vi "write_metadata_attributes.vi"(5 "Group ID":string, 6 "error in (no error)":errorcluster, 8 "Cluster":T1 {"File Location" items=["Unknown"=-5, "IDL Processing"=-4, "Writing from Queue"=-3, "Labview Files"=-2, "Retry Labview files"=-1, "Local Cache "=0, "Storage"=1]; "Estimate Source" items=["Any Source."=-2, "No Shot"=-1, "Basic Labview Estimate"=0, "IDL Estimate From Andrew"=1, "IDL Estimate From Tobin"=2, "Old Metadata"=3]}, 9 "group ref":i32) -> (0 "error out":errorcluster, 3 "group ref out":i32)   [LabVIEW 2013]
uses:
  Public API/Query_Dust_Event.ctl
  Controls/Estimate_source.ctl
  Controls/File_location.ctl
  <vilib>/addons/h5labview/H5Attrib.lvlib
panel:
  # "Dust Event"
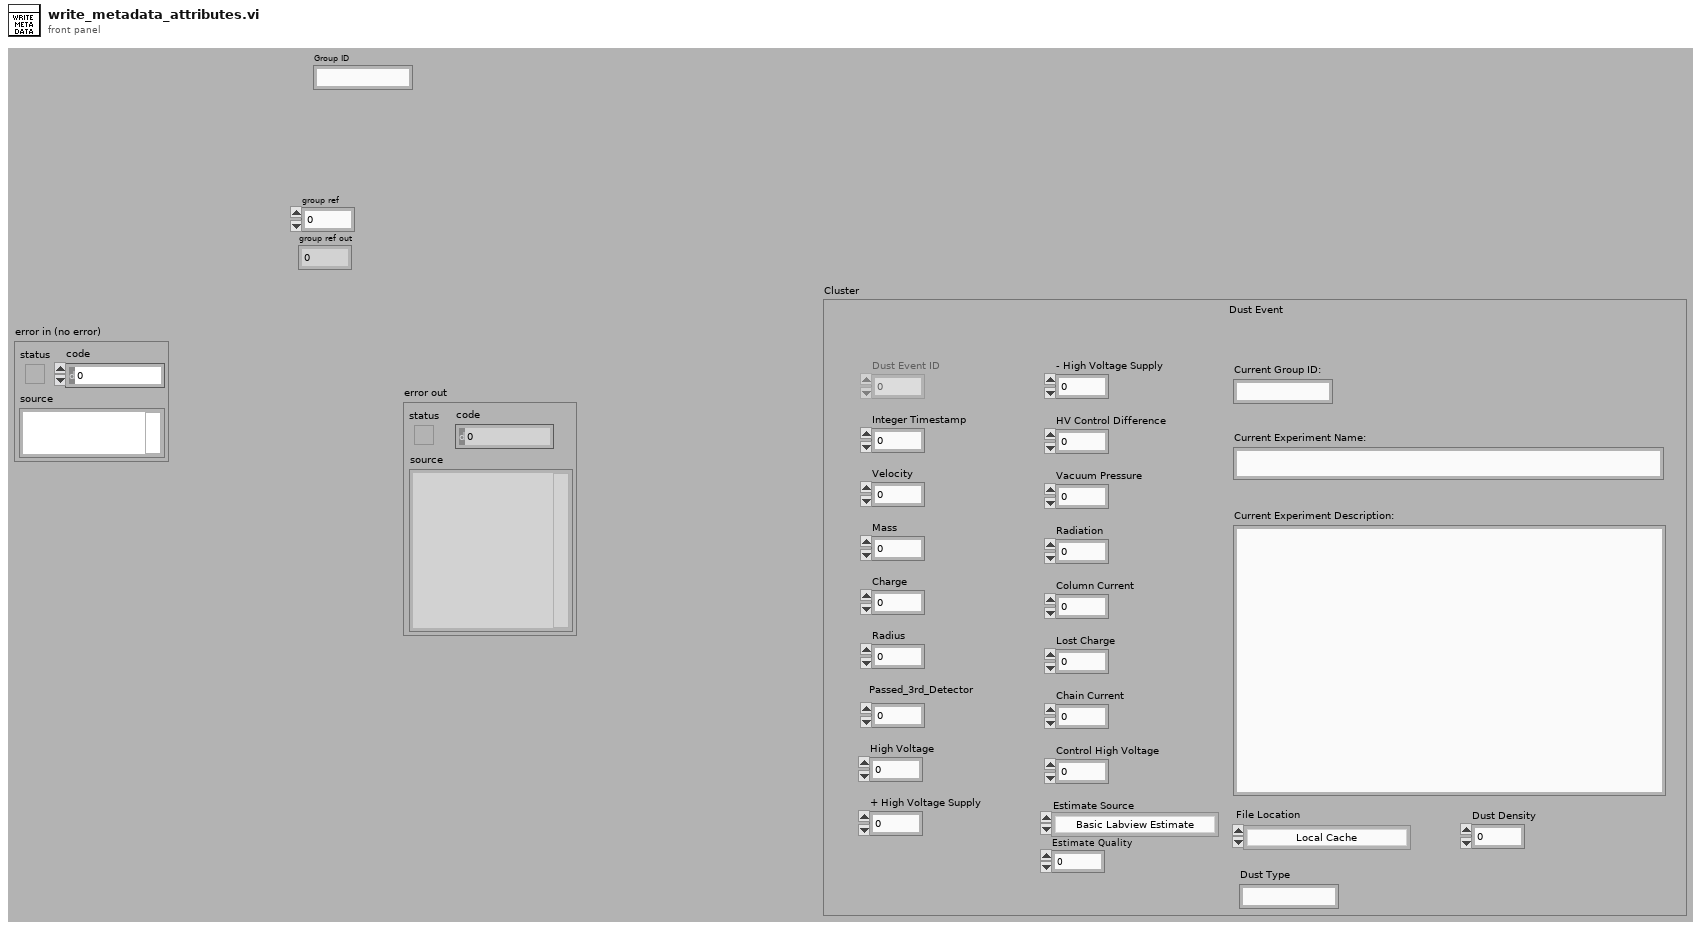
[diagram p1: front panel]
types:
  T1 = typedef "Query_Dust_Event.ctl" = cluster{"Dust Event ID":i64, "Integer Timestamp":i64, "Velocity":sgl, "Mass":sgl, "Charge":sgl, "Radius":sgl, "Passed_3rd_Detector":i8, "High Voltage":sgl, "+ High Voltage Supply":sgl, "- High Voltage Supply":sgl, "HV Control Difference":sgl, "Vacuum Pressure":sgl, "Radiation":sgl, "Column Current":sgl, "Lost Charge":sgl, "Chain Current":sgl, "Control High Voltage":sgl, "Current Group ID:":string, "Current Experiment Name:":string, "Current Experiment Description:":string, "Estimate Source":T2, "Estimate Quality":sgl, "File Location":T3, "Dust Type":string, "Dust Density":sgl}
  T2 = typedef "Estimate_source.ctl" = i8
  T3 = typedef "File_location.ctl" = i8
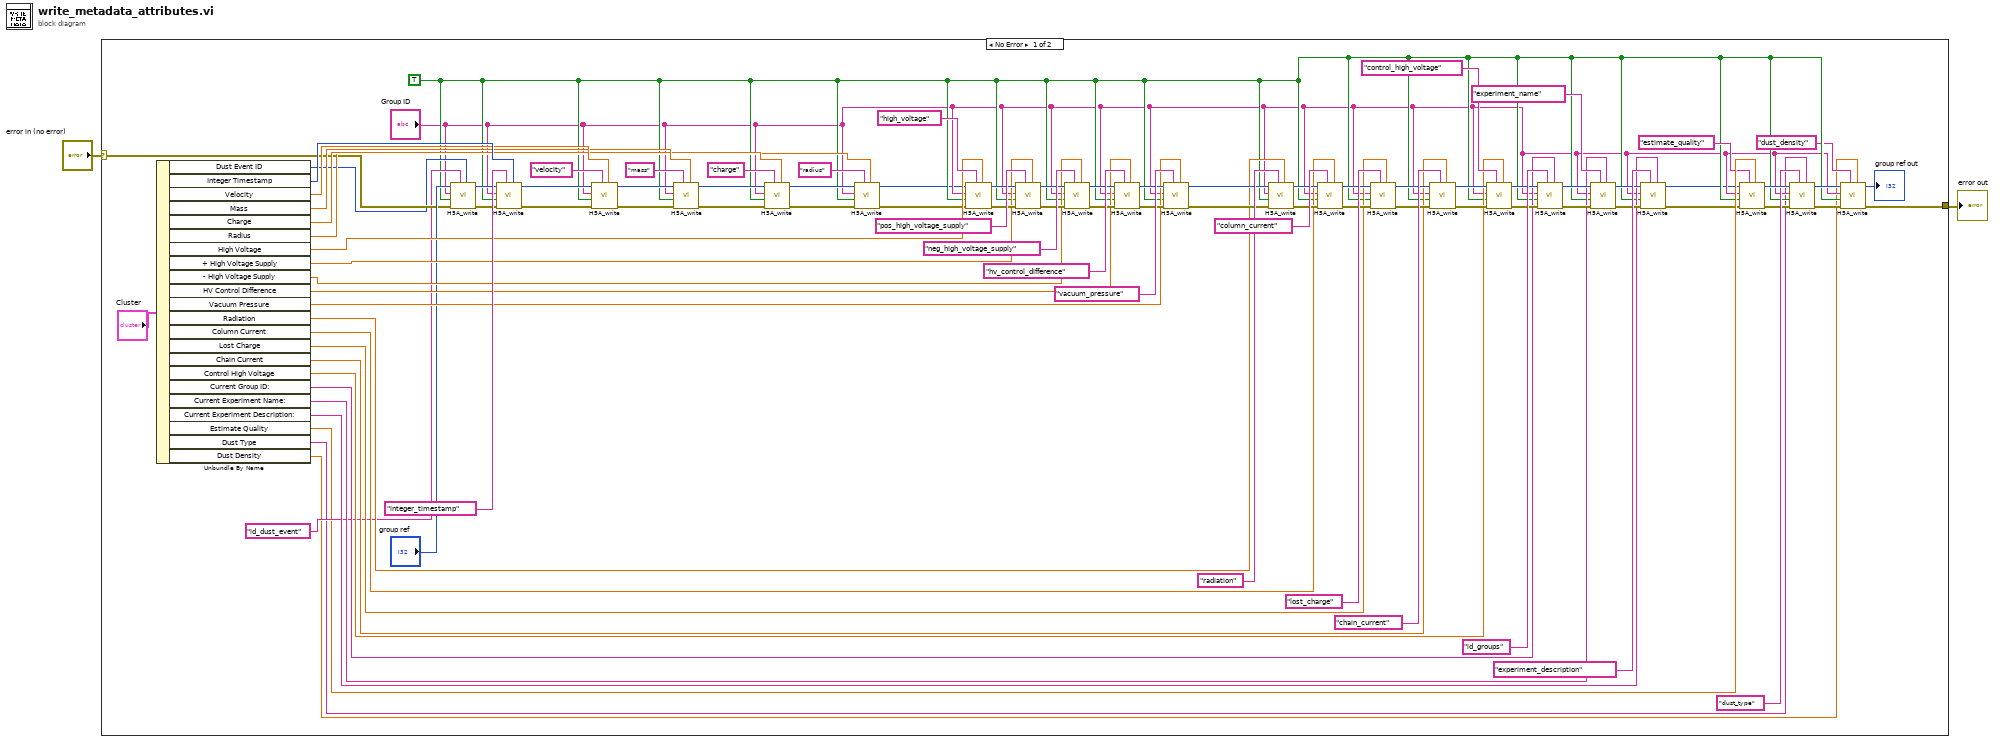
[diagram p0: block diagram]
diagram:
  n1 = case shown="No Error" "error in (no error)" {
    selector: "error in (no error)" -> [w23 w96]
    tunnel: [w13 w96] -> w1
    frame No Error {
      w11 = TRUE
      n2 = Unbundle By Name("Cluster") -> ("Dust Event ID"=w22:i64, "Integer Timestamp"=w94:i64, "Velocity"=w92:sgl, "Mass"=w86:sgl, "Charge"=w41:sgl, "Radius"=w40:sgl, "High Voltage"=w39:sgl, "+ High Voltage Supply"=w38:sgl, "- High Voltage Supply"=w37:sgl, "HV Control Difference"=w36:sgl, "Vacuum Pressure"=w35:sgl, "Radiation"=w34:sgl, "Column Current"=w33:sgl, "Lost Charge"=w32:sgl, "Chain Current"=w31:sgl, "Control High Voltage"=w30:sgl, "Current Group ID:"=w29:string, "Current Experiment Name:"=w28:string, "Current Experiment Description:"=w27:string, "Estimate Quality"=w20:sgl, "Dust Type"=w9:string, "Dust Density"=w7:sgl)
      n3 = call <vilib>:"H5A_write.vi"("value"=w22, "attrib_name"="id_dust_event", "error in (no error)"=w23, "overwrite? (F)"=w11, "obj_name"="Group ID", "ref"="group ref") -> ("error out"=w24:errorcluster, "ref out"=w26:i32)  [unwired: 2 in]
      n4 = call <vilib>:"H5A_write.vi"("value"=w94, "attrib_name"="integer_timestamp", "error in (no error)"=w24, "overwrite? (F)"=w11, "obj_name"="Group ID", "ref"=w26) -> ("error out"=w90:errorcluster, "ref out"=w91:i32)  [unwired: 2 in]
      n5 = call <vilib>:"H5A_write.vi"("value"=w92, "attrib_name"="velocity", "error in (no error)"=w90, "overwrite? (F)"=w11, "obj_name"="Group ID", "ref"=w91) -> ("error out"=w88:errorcluster, "ref out"=w89:i32)  [unwired: 2 in]
      n6 = call <vilib>:"H5A_write.vi"("value"=w86, "attrib_name"="mass", "error in (no error)"=w88, "overwrite? (F)"=w11, "obj_name"="Group ID", "ref"=w89) -> ("error out"=w70:errorcluster, "ref out"=w85:i32)  [unwired: 2 in]
      n7 = call <vilib>:"H5A_write.vi"("value"=w41, "attrib_name"="charge", "error in (no error)"=w70, "overwrite? (F)"=w11, "obj_name"="Group ID", "ref"=w85) -> ("error out"=w69:errorcluster, "ref out"=w54:i32)  [unwired: 2 in]
      n8 = call <vilib>:"H5A_write.vi"("value"=w40, "attrib_name"="radius", "error in (no error)"=w69, "overwrite? (F)"=w11, "obj_name"="Group ID", "ref"=w54) -> ("error out"=w4:errorcluster, "ref out"=w3:i32)  [unwired: 2 in]
      n9 = call <vilib>:"H5A_write.vi"("value"=w39, "attrib_name"="high_voltage", "error in (no error)"=w4, "overwrite? (F)"=w11, "obj_name"="Group ID", "ref"=w3) -> ("error out"=w68:errorcluster, "ref out"=w53:i32)  [unwired: 2 in]
      n10 = call <vilib>:"H5A_write.vi"("value"=w38, "attrib_name"="pos_high_voltage_supply", "error in (no error)"=w68, "overwrite? (F)"=w11, "obj_name"="Group ID", "ref"=w53) -> ("error out"=w67:errorcluster, "ref out"=w52:i32)  [unwired: 2 in]
      n11 = call <vilib>:"H5A_write.vi"("value"=w37, "attrib_name"="neg_high_voltage_supply", "error in (no error)"=w67, "overwrite? (F)"=w11, "obj_name"="Group ID", "ref"=w52) -> ("error out"=w66:errorcluster, "ref out"=w51:i32)  [unwired: 2 in]
      n12 = call <vilib>:"H5A_write.vi"("value"=w36, "attrib_name"="hv_control_difference", "error in (no error)"=w66, "overwrite? (F)"=w11, "obj_name"="Group ID", "ref"=w51) -> ("error out"=w65:errorcluster, "ref out"=w50:i32)  [unwired: 2 in]
      n13 = call <vilib>:"H5A_write.vi"("value"=w35, "attrib_name"="vacuum_pressure", "error in (no error)"=w65, "overwrite? (F)"=w11, "obj_name"="Group ID", "ref"=w50) -> ("error out"=w64:errorcluster, "ref out"=w49:i32)  [unwired: 2 in]
      n14 = call <vilib>:"H5A_write.vi"("value"=w34, "attrib_name"="radiation", "error in (no error)"=w64, "overwrite? (F)"=w11, "obj_name"="Group ID", "ref"=w49) -> ("error out"=w63:errorcluster, "ref out"=w48:i32)  [unwired: 2 in]
      n15 = call <vilib>:"H5A_write.vi"("value"=w33, "attrib_name"="column_current", "error in (no error)"=w63, "overwrite? (F)"=w11, "obj_name"="Group ID", "ref"=w48) -> ("error out"=w62:errorcluster, "ref out"=w47:i32)  [unwired: 2 in]
      n16 = call <vilib>:"H5A_write.vi"("value"=w32, "attrib_name"="lost_charge", "error in (no error)"=w62, "overwrite? (F)"=w11, "obj_name"="Group ID", "ref"=w47) -> ("error out"=w61:errorcluster, "ref out"=w46:i32)  [unwired: 2 in]
      n17 = call <vilib>:"H5A_write.vi"("value"=w31, "attrib_name"="chain_current", "error in (no error)"=w61, "overwrite? (F)"=w11, "obj_name"="Group ID", "ref"=w46) -> ("error out"=w60:errorcluster, "ref out"=w45:i32)  [unwired: 2 in]
      n18 = call <vilib>:"H5A_write.vi"("value"=w30, "attrib_name"="control_high_voltage", "error in (no error)"=w60, "overwrite? (F)"=w11, "obj_name"="Group ID", "ref"=w45) -> ("error out"=w59:errorcluster, "ref out"=w44:i32)  [unwired: 2 in]
      n19 = call <vilib>:"H5A_write.vi"("value"=w29, "attrib_name"="id_groups", "error in (no error)"=w59, "overwrite? (F)"=w11, "obj_name"="Group ID", "ref"=w44) -> ("error out"=w58:errorcluster, "ref out"=w43:i32)  [unwired: 2 in]
      n20 = call <vilib>:"H5A_write.vi"("value"=w28, "attrib_name"="experiment_name", "error in (no error)"=w58, "overwrite? (F)"=w11, "obj_name"="Group ID", "ref"=w43) -> ("error out"=w56:errorcluster, "ref out"=w42:i32)  [unwired: 2 in]
      n21 = call <vilib>:"H5A_write.vi"("value"=w27, "attrib_name"="experiment_description", "error in (no error)"=w56, "overwrite? (F)"=w11, "obj_name"="Group ID", "ref"=w42) -> ("error out"=w6:errorcluster, "ref out"=w5:i32)  [unwired: 2 in]
      n22 = call <vilib>:"H5A_write.vi"("value"=w20, "attrib_name"="estimate_quality", "error in (no error)"=w6, "overwrite? (F)"=w11, "obj_name"="Group ID", "ref"=w5) -> ("error out"=w12:errorcluster, "ref out"=w18:i32)  [unwired: 2 in]
      n23 = call <vilib>:"H5A_write.vi"("value"=w9, "attrib_name"="dust_type", "error in (no error)"=w12, "overwrite? (F)"=w11, "obj_name"="Group ID", "ref"=w18) -> ("error out"=w14:errorcluster, "ref out"=w17:i32)  [unwired: 2 in]
      n24 = call <vilib>:"H5A_write.vi"("value"=w7, "attrib_name"="dust_density", "error in (no error)"=w14, "overwrite? (F)"=w11, "obj_name"="Group ID", "ref"=w17) -> ("error out"=w13:errorcluster, "ref out"=→"group ref out":i32)  [unwired: 2 in]
    }
    frame Error {
    }
  }
  "error out" <- w1
